vi "FindItemByTag.vi"(8 "error in (no error)":errorcluster, 10 "Tag":string, 11 "MenuStrip in":refnum<class "MGI_MenuStrip.lvclass">) -> (0 "error out":errorcluster, 2 "Tool Strip Menu Item":refnum<k24>, 3 "MenuStrip out":refnum<class "MGI_MenuStrip.lvclass">)   [LabVIEW 2016, in "MGI_MenuStrip.lvclass"]
doc: "Authored by Derek E. Trepanier\nsupport@mooregoodideas.com\nwww.mooregoodideas.com\n\nCopyright (c) 2012, Moore Good Ideas, Inc.\n\nAll rights reserved.\n\nRedistribution and use in source and binary forms, with or without modification, are permitted provided that the following conditions are met:\n\n * Redistributions of source code must retain the above copyright notice, this list of conditions and the following disclaimer.\n * Redistributions in binary form must reproduce the above copyright notice, this list of conditions and the following disclaimer in the documentation and/or other materials provided with the distribution.\n * Neither the name of Moore Good Ideas, Inc. nor the names of its contributors may be used to endorse or promote products derived from this software without specific prior written permission.\n\nTHIS SOFTWARE IS PROVIDED BY THE COPYRIGHT HOLDERS AND CONTRIBUTORS \"AS IS\" AND ANY EXPRESS OR IMPLIED WARRANTIES, INCLUDING, BUT NOT LIMITED TO, THE IMPLIED WARRANTIES OF MERCHANTABILITY AND FITNESS FOR A PARTICULAR PURPOSE ARE DISCLAIMED. IN NO EVENT SHALL THE COPYRIGHT OWNER OR CONTRIBUTORS BE LIABLE FOR ANY DIRECT, INDIRECT, INCIDENTAL, SPECIAL, EXEMPLARY, OR CONSEQUENTIAL DAMAGES (INCLUDING, BUT NOT LIMITED TO, PROCUREMENT OF SUBSTITUTE GOODS OR SERVICES; LOSS OF USE, DATA, OR PROFITS; OR BUSINESS INTERRUPTION) HOWEVER CAUSED AND ON ANY THEORY OF LIABILITY, WHETHER IN CONTRACT, STRICT LIABILITY, OR TORT (INCLUDING NEGLIGENCE OR OTHERWISE) ARISING IN ANY WAY OUT OF THE USE OF THIS SOFTWARE, EVEN IF ADVISED OF THE POSSIBILITY OF SUCH DAMAGE."
uses:
  <userlib>/_MGI/Menu Building/MenuTypes/MenuStrip/MGI_MenuStrip.lvclass
  System.Windows.Forms
  <userlib>/_MGI/Menu Building/MenuTypes/MenuStrip/MGI_MenuStrip.lvclass/MGI_MenuStrip.ctl
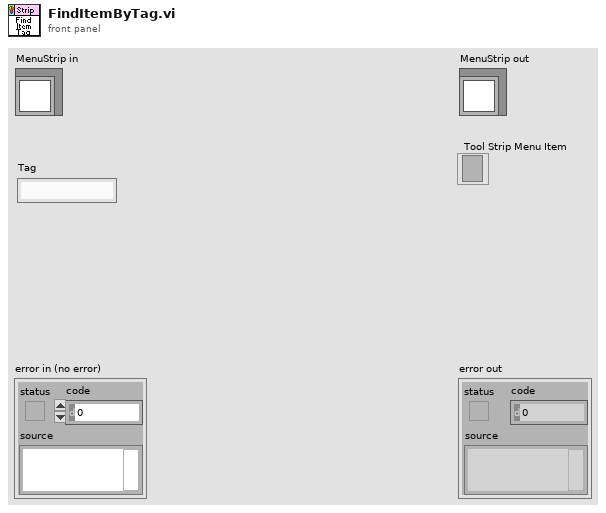
[diagram p1: front panel]
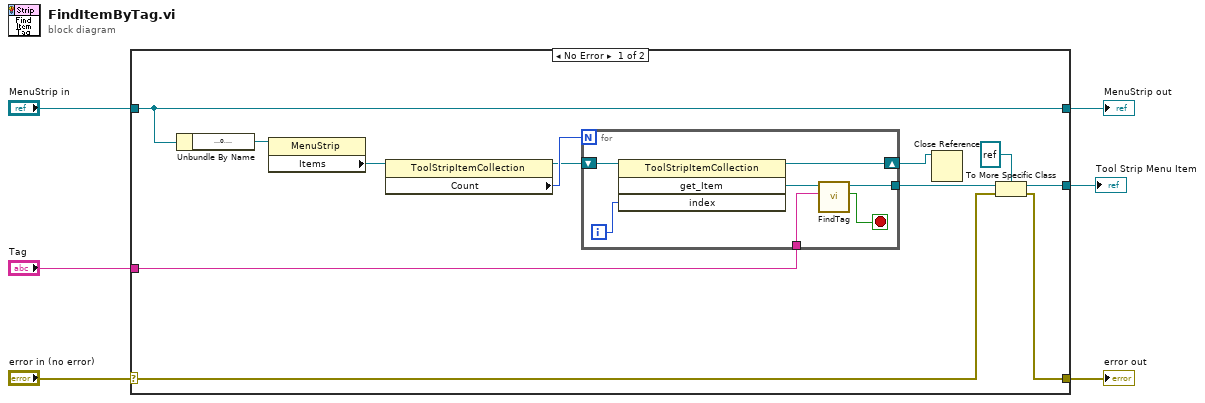
[diagram p0: block diagram]
diagram:
  n1 = case shown="No Error" "error in (no error)" {
    selector: "error in (no error)" -> [w9 w27]
    tunnel: [w8 w27] -> w5
    tunnel: [w18 w26] -> w3
    tunnel: "MenuStrip in" -> [w18 w26]
    tunnel: "Tag" -> [w13 _]
    tunnel: [w11 _] -> w1
    frame No Error {
      n2 = Unbundle By Name(w18) -> ("MenuStrip"=w17:refnum<k24>)
      n3 = property class="MenuStrip"(reference=w17) -> ("Items"=w16:refnum<k24>)  [unwired: 1 in, 2 out]
      n4 = property class="ToolStripItemCollection"(reference=w16) -> (reference out=w14:refnum<k24>, "Count"=w15:i32)  [unwired: 1 in, 1 out]
      n5 = for {
        N: w15 -> [_]
        tunnel: w13 -> [w21]
        tunnel: [w20] -> w12
        shift-right: [w19] -> w7
        shift-left: w14 -> [w25]
        i -> [w24]
        stop <- w22 stop-if-true
        n6 = invoke class="ToolStripItemCollection" method="get_Item"(reference=w25, "index"=w24) -> (reference out=w19:refnum<k24>, "get_Item"=w23:refnum<k24>)  [unwired: 2 in, 2 out]
        n7 = call <userlib>:"FindTag.vi"("Tag"=w21, "ToolStripItem"=w23) -> ("Found"=w22:bool, "ToolStripItem out"=w20:refnum<k24>)  [unwired: 7 in, 1 out]
      }
      n8 = Close Reference(reference=w7) -> ()  [unwired: 1 in, 1 out]
      n9 = To More Specific Class(target class=refnum<k24> refnum ("new reference"), reference=w12, error in=w9) -> (specific class reference=w11:refnum<k24>, error out=w8:errorcluster)
    }
    frame Error {
    }
  }
  "error out" <- w5
  "MenuStrip out" <- w3
  "Tool Strip Menu Item" <- w1
